vi "Update QuickDrop ShortCuts Hints.vi"() -> ()   [LabVIEW 2020, in "NEVSTOP_QuickDrop.lvlib"]
uses:
  NEVSTOP_QuickDrop.lvlib
  <resource>/dialog/lvconfig.llb/LV Config Read String.vi
panel:
  out "value":string
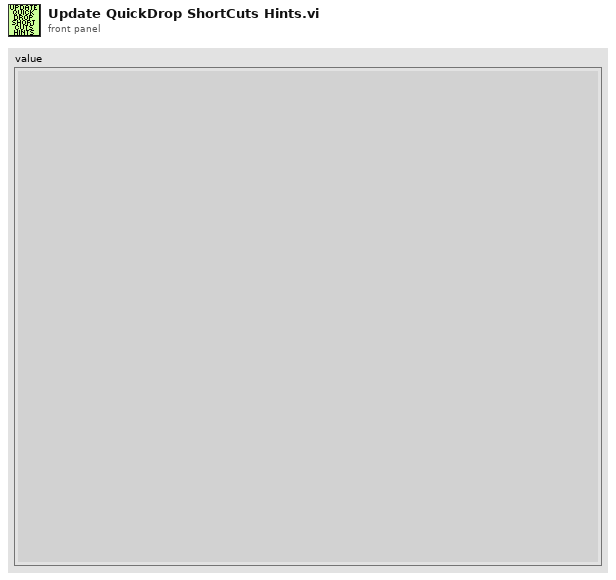
[diagram p1: front panel]
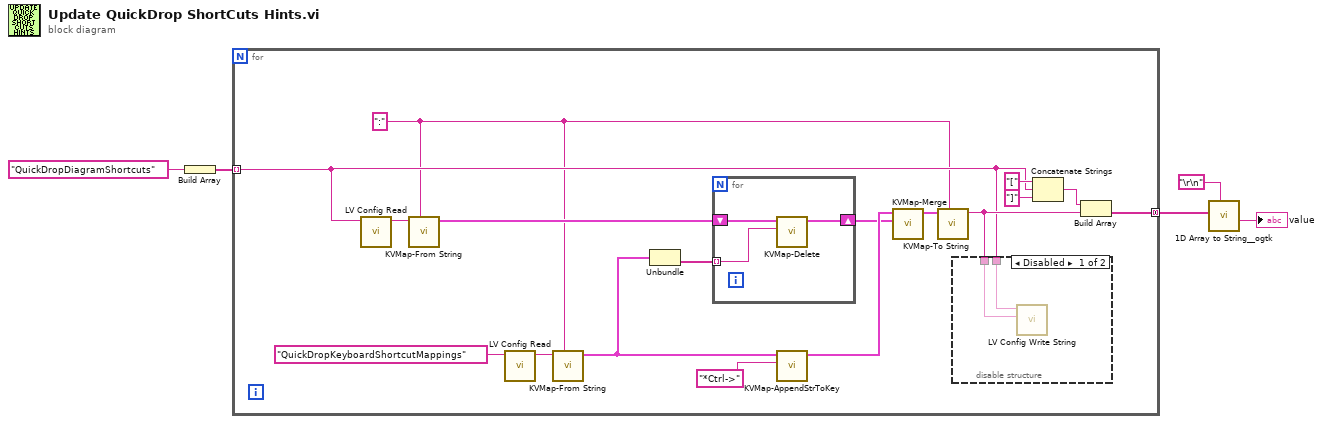
[diagram p0: block diagram]
diagram:
  n1 = Build Array("QuickDropDiagramShortcuts" ("key")) -> (w4:string[])
  n2 = for {
    tunnel: w4 -> [w7] mode=indexing
    tunnel: [w8] -> w2 mode=concatenating
    w6 = ":" ("delimiter (Tab)")
    n3 = call-poly <resource>:"LV Config Read.vi"("key"=w7) -> ("value"=w20:string)  [unwired: 4 in, 2 out]
    n4 = call "KVMap-From String.vi"("delimiter (Tab)"=w6, "value"=w20) -> ("Cluster"=w19:cluster{string[], string[]})  [unwired: 9 in]
    n5 = call-poly <resource>:"LV Config Read.vi"("key"="QuickDropKeyboardShortcutMappings") -> ("value"=w21:string)  [unwired: 4 in, 2 out]
    n6 = call "KVMap-From String.vi"("delimiter (Tab)"=w6, "value"=w21) -> ("Cluster"=w17:cluster{string[], string[]})  [unwired: 9 in]
    n7 = Unbundle(w17) -> (w16:string[])  [unwired: 1 out]
    n8 = for {
      shift-right: [w26] -> w14
      shift-left: w19 -> [w27]
      tunnel: w16 -> [w25] mode=indexing
      n9 = call "KVMap-Delete.vi"("element"=w25, "Cluster in"=w27) -> ("Cluster out"=w26:cluster{string[], string[]})  [unwired: 9 in]
    }
    n10 = call "KVMap-AppendStrToKey.vi"("string"="*Ctrl->", "Cluster in"=w17) -> ("Cluster out"=w15:cluster{string[], string[]})  [unwired: 9 in]
    n11 = call "KVMap-Merge.vi"("Cluster 2"=w14, "Cluster in"=w15) -> ("Cluster"=w13:cluster{string[], string[]})  [unwired: 8 in]
    n12 = call "KVMap-To String.vi"("string"=w6, "Cluster"=w13) -> ("value"=w9:string)  [unwired: 9 in]
    n13 = disable-structure shown="Disabled" {
      disable-tunnel: w9 -> [w24 _]
      disable-tunnel: w7 -> [w23 _]
      frame Disabled {
        n14 = call <resource>:"LV Config Write String.vi"("value"=w24, "key"=w23) -> ()  [unwired: 5 in, 1 out]
      }
      frame Enabled {
      }
    }
    n15 = Concatenate Strings("[" ("string"), w7, "]" ("string")) -> (w12:string)
    n16 = Build Array(w12, w9) -> (w8:string[])
  }
  n17 = call <userlib>:"1D Array to String__ogtk.vi"("delimiter (Tab)"="\r\n", "Array of Strings"=w2) -> ("delimited string"=→"value":string)  [unwired: 9 in]
